vi "constructor.vi"(8 "error in (no error)":errorcluster) -> (0 "error out":errorcluster, 3 "HWConfiguration out":refnum<class "HWConfigurations.lvclass">)   [LabVIEW 2009, in "Tools.lvlib" / "DatabaseHelpers.lvlib" / "HWConfigurations.lvclass"]
uses:
  HWConfigurations.lvclass
  XmlParser.lvclass
  Filing/FileSystem/FileSystem.lvclass
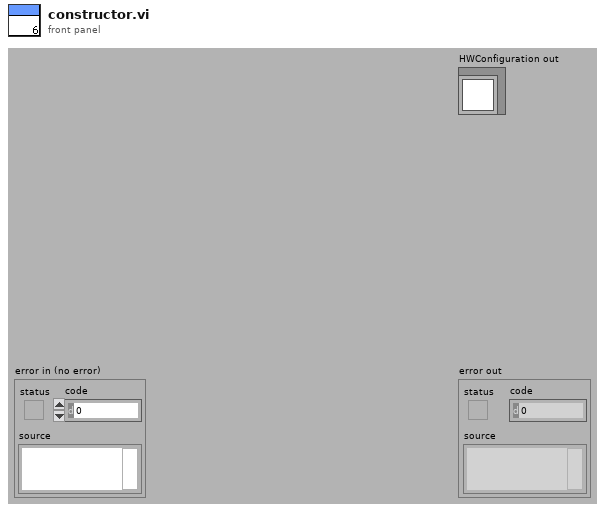
[diagram p1: front panel]
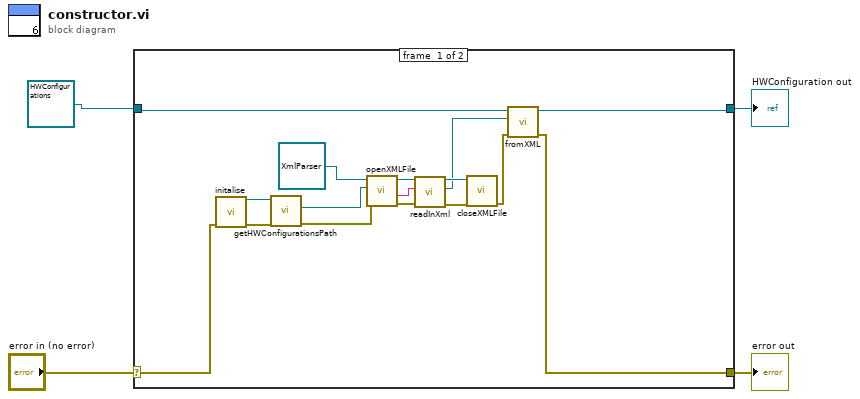
[diagram p0: block diagram]
diagram:
  n1 = case shown="No Error" "error in (no error)" {
    selector: "error in (no error)" -> [w9 w22]
    tunnel: [w5 w22] -> w3
    tunnel: [w19 w21] -> w2
    tunnel: refnum<class "HWConfigurations.lvclass"> refnum ("Tools.lvlib:DatabaseHelpers.lvlib:HWConfiguration.lvclass") -> [w20 w21]
    frame #0 {
      n2 = call "initalise.vi"("error in (no error)"=w9) -> ("error out"=w10:errorcluster, "FileSystem out"=w11:refnum<class "FileSystem.lvclass">)  [unwired: 9 in]
      n3 = call "getHWConfigurationsPath.vi"("error in (no error)"=w10, "FileSystem.lvclass in"=w11) -> ("error out"=w7:errorcluster, "HWConfigurations"=w12:path)  [unwired: 7 in, 1 out]
      n4 = call "openXMLFile.vi"("error in (no error)"=w7, "Path"=w12, "XmlParser in"=refnum<class "XmlParser.lvclass"> refnum) -> ("error out"=w13:errorcluster, "xmlFileInput"=w14:string, "XmlParser out"=w18:refnum<class "XmlParser.lvclass">)  [unwired: 6 in]
      n5 = call "readInXml.vi"("error in (no error)"=w13, "xmlString"=w14, "XmlParser in"=w18) -> ("error out"=w16:errorcluster, "xmlNode"=w15:refnum<class "xmlNode.lvclass">, "XmlParser out"=w17:refnum<class "XmlParser.lvclass">)  [unwired: 6 in]
      n6 = call-dynamic "closeXMLFile.vi"("error in (no error)"=w16, "XmlParser in"=w17) -> ("error out"=w6:errorcluster)  [unwired: 8 in, 1 out]
      n7 = call "fromXML.vi"("error in (no error)"=w6, "xmlNode"=w15, "HWConfiguration in"=w20) -> ("error out"=w5:errorcluster, "HWConfiguration out"=w19:refnum<class "HWConfigurations.lvclass">)  [unwired: 7 in]
    }
    frame #1 {
    }
  }
  "error out" <- w3
  "HWConfiguration out" <- w2
